vi "Get SMO Name.vi"(8 "error in (no error)":errorcluster, 11 "Inst.TC in":refnum<class "Inst.TC.lvclass">) -> (0 "error out":errorcluster, 2 "SMO Name":string, 3 "Inst.TC out":refnum<class "Inst.TC.lvclass">)   [LabVIEW 2019, in "Inst.TC.lvclass"]
uses:
  Inst.TC.lvclass
  <userlib>/LevyLab/Instrument Framework/Instrument Types/Cryostat/Instrument.Cryostat.lvclass
  b29bc2d5-5107-4929-bcf9-f3c2a96a48cd.vi
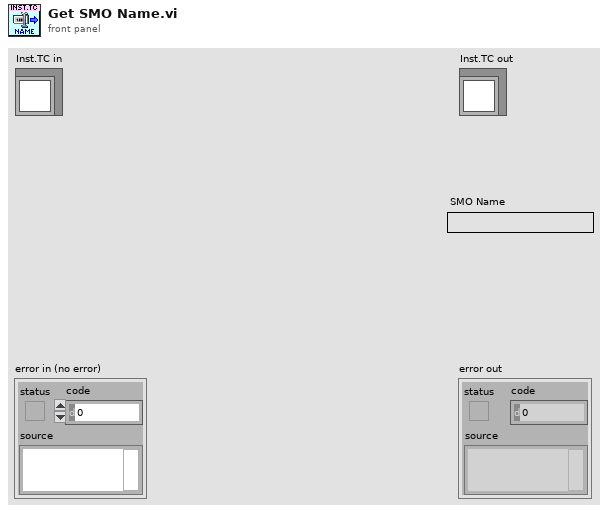
[diagram p1: front panel]
types:
  T1 = typedef "Inst.TC.lvclass/Inst.TC.Type--Enum.ctl" = enum16{"CF.TC", "CF.TC.Z", "CF.FP", "MNK.TC", "MNK.TC.Z", "MNK.FP"}
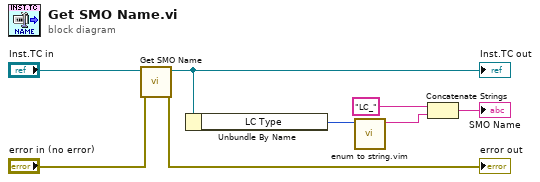
[diagram p0: block diagram]
diagram:
  n1 = call-parent "Get SMO Name.vi"("error in (no error)"="error in (no error)", "Instrument in"="Inst.TC in") -> ("error out"=→"error out":errorcluster, "Instrument out"=w4:refnum<class "Inst.TC.lvclass">)  [unwired: 7 in, 1 out]
  "Inst.TC out" <- w4
  n2 = Unbundle By Name(w4) -> ("LC Type"=w6:T1)
  n3 = call "enum to string.vim"("enum in"=w6) -> ("string out"=w5:string)  [unwired: 9 in, 1 out]
  n4 = Concatenate Strings("LC_" ("SMO Name"), w5) -> (→"SMO Name":string)
